vi "GFITS_getKeyvalueFromDBSHandler2.vi"(0 "key name in header":string, 1 "Database RefNum in":T3, 2 "action":enum16{"get", "clear"}(ring), 3 "extension":i32, 5 "varname":string, 7 "comment":string, 11 "error in (no error)":errorcluster, 12 "nd queue":bool, 13 "expID in":string) -> (6 "table out":string[][](table), 8 "expID":string, 10 "datatype":u16[](array[numeric]), 14 "function to use":string, 15 "error out":errorcluster)   [LabVIEW 2016]
uses:
  GFITS_datatypesctl.ctl
  DBSHAND/private/vis/DatabaseHand_RefNum.ctl
  DBSHAND/private/vis/DatabaseHand_Element_Get(3DArr).vi
  DBSHAND/private/vis/DatabaseHand_Element_Get(1DArr).vi
  DBSHAND/private/vis/DatabaseHand_Element_Get(string).vi
panel:
  out "Array":T1(array[cluster])
  in  "key":T2
  in  "Types":T4={"TBIT"=1, "TBYTE"=11, "TSTRING"=16, "TSHORT"=21, "TLONG"=41, "TFLOAT"=42, "TDOUBLE"=82, "TCOMPLEX"=83, "TDBLCOMPLEX"=163, "TUINT"=30, "TUSHORT"=20, "TULONG"=40, "TINT"=31, "TSBYTE"=12, "TLONGLONG"=81, "TLOGICAL"=14}
  in  "Supported DataTypes":i32(listbox)
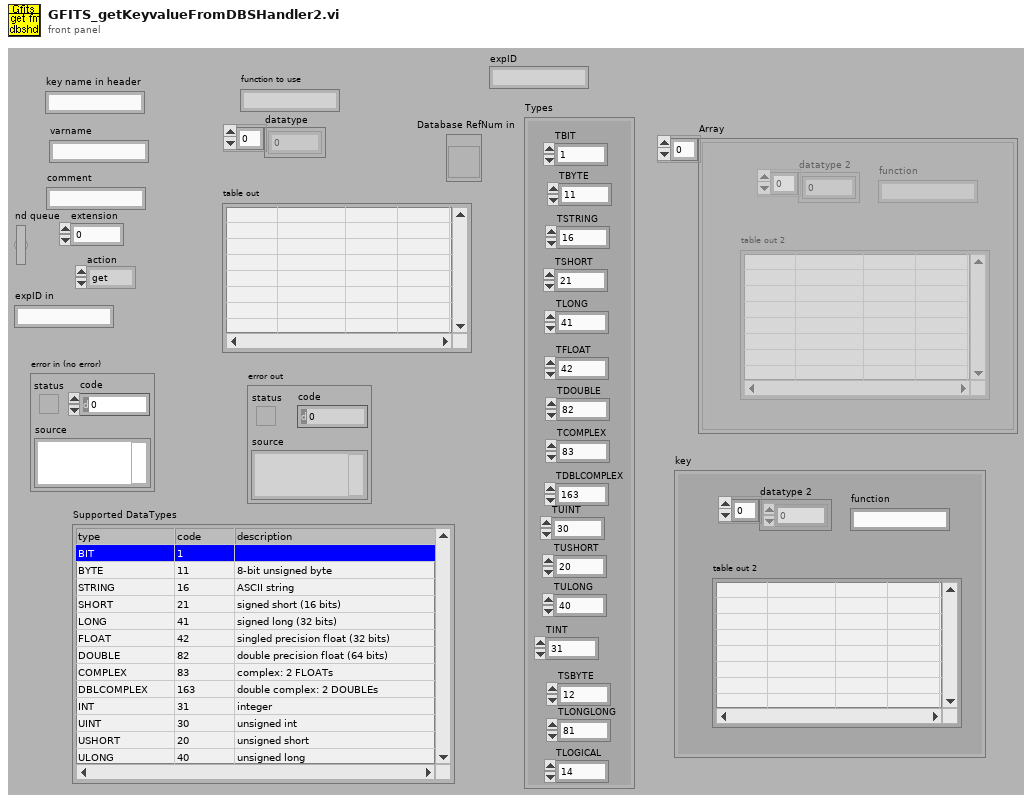
[diagram p1: front panel]
types:
  T1 = cluster{"table out 2":string[][], "datatype 2":u16[], "function":string}[]
  T2 = cluster{"table out 2":string[][], "datatype 2":u16[], "function":string}
  T3 = typedef "DatabaseHand_RefNum.ctl" = refnum<vi>
  T4 = typedef "GFITS_datatypesctl.ctl" = cluster{"TBIT":i32, "TBYTE":i32, "TSTRING":i32, "TSHORT":i32, "TLONG":i32, "TFLOAT":i32, "TDOUBLE":i32, "TCOMPLEX":i32, "TDBLCOMPLEX":i32, "TUINT":i32, "TUSHORT":i32, "TULONG":i32, "TINT":i32, "TSBYTE":i32, "TLONGLONG":i32, "TLOGICAL":i32}
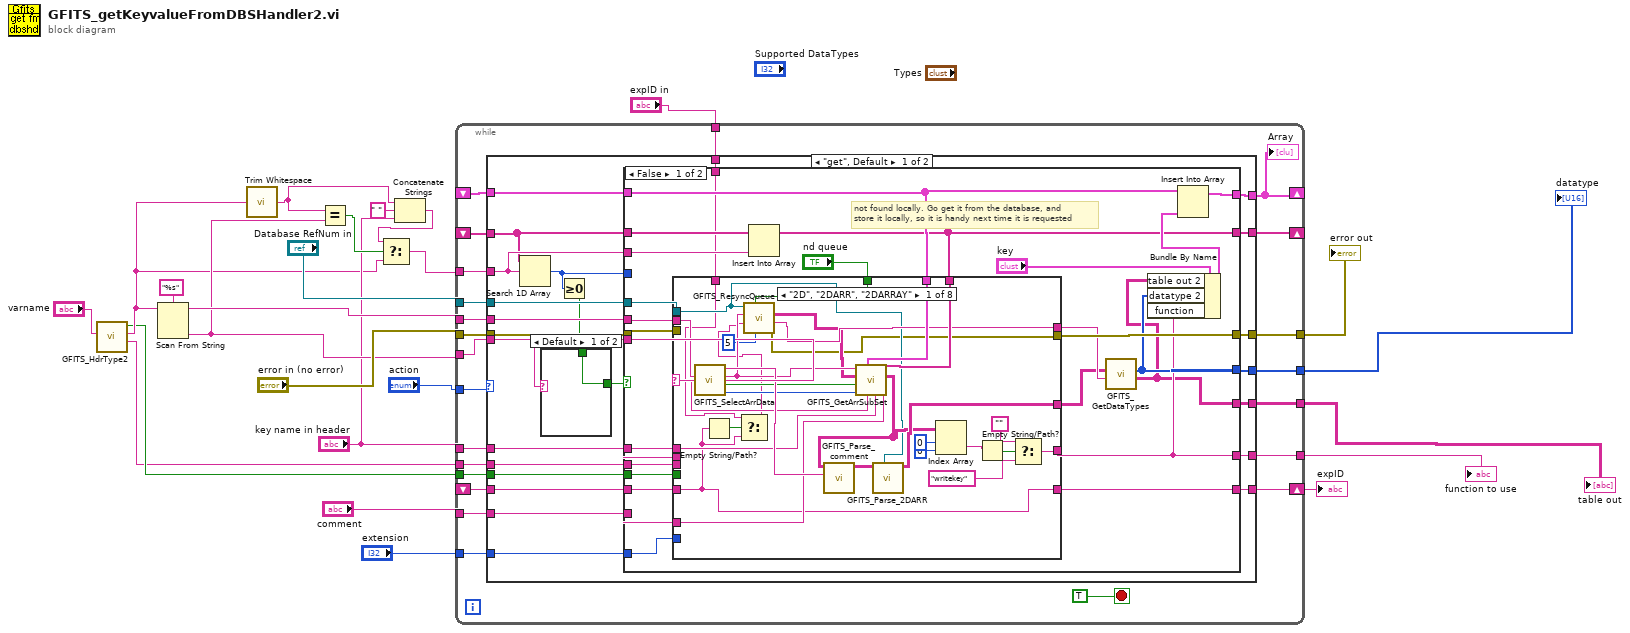
[diagram p0: block diagram]
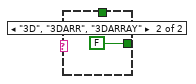
[diagram p2: hidden frame]
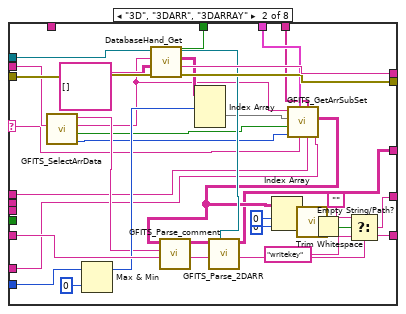
[diagram p3: hidden frame]
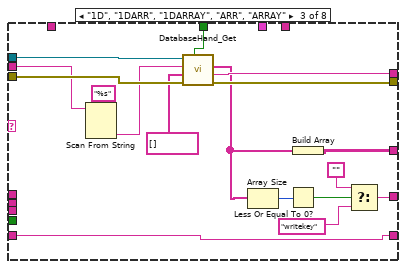
[diagram p4: hidden frame]
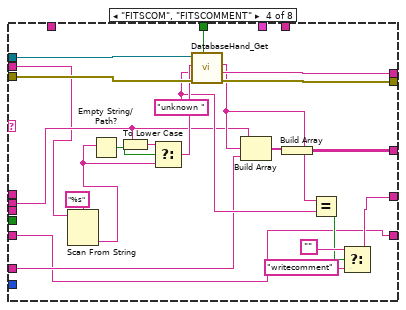
[diagram p5: hidden frame]
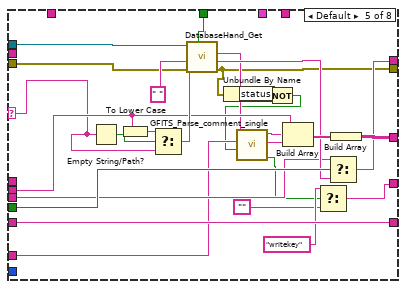
[diagram p6: hidden frame]
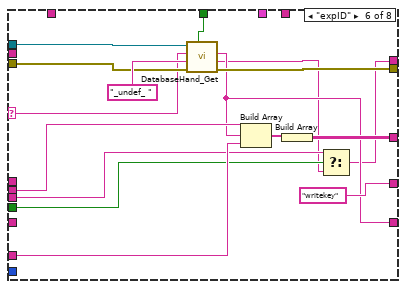
[diagram p7: hidden frame]
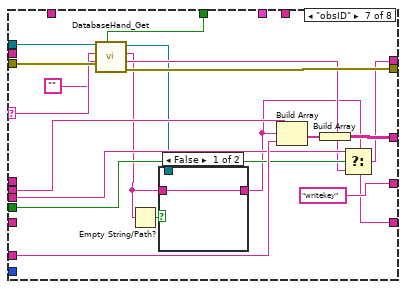
[diagram p8: hidden frame]
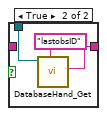
[diagram p9: hidden frame]
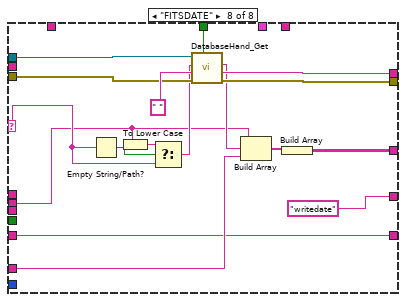
[diagram p10: hidden frame]
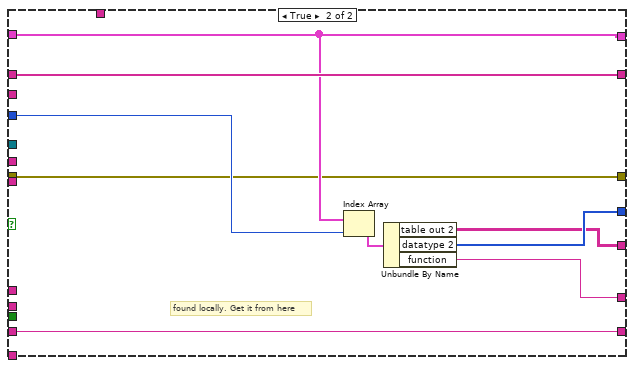
[diagram p11: hidden frame]
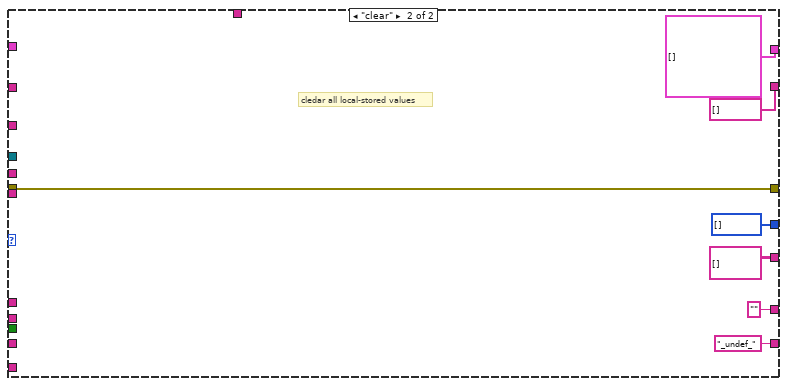
[diagram p12: hidden frame]
diagram:
  n1 = call "GFITS_HdrType2.vi"("keyval"="varname") -> ("type"=w2:string, "keyval out"=w4:string, "specified"=w3:bool)  [unwired: 8 out]
  n2 = Scan From String(format string="%s", input string=w4) -> (remaining string=w21:string, output 1=w14:string)  [unwired: 2 in, 3 out]
  n3 = call <vilib>:"Trim Whitespace.vi"("string"=w4) -> ("trimmed string"=w12:string)  [unwired: 1 in]
  n4 = Equal?(x=w12, y=w14) -> (x = y?=w13:bool)
  n5 = Concatenate Strings(w12, " " ("string"), "key name in header") -> (w9:string)
  n6 = Select(t=w9, s=w13, f=w4) -> (s? t:f=w8:string)
  n7 = while {
    tunnel: "Database RefNum in" -> [w47]
    tunnel: "error in (no error)" -> [w46]
    tunnel: w14 -> [w45]
    tunnel: w21 -> [w44]
    tunnel: [w43] -> w20
    tunnel: "key name in header" -> [w42]
    tunnel: "comment" -> [w41]
    tunnel: [w40] -> w19
    tunnel: [w39] -> w15
    shift-right: [w34] -> _
    shift-left: _ -> [w33]
    tunnel: "action" -> [w37]
    shift-right: [w31] -> _
    shift-left: _ -> [w32]
    tunnel: [w36] -> w17
    tunnel: w8 -> [w35]
    shift-right: [w30] -> w7
    shift-left: _ -> [w29]
    tunnel: "extension" -> [w28]
    tunnel: w3 -> [w27]
    tunnel: w2 -> [w26]
    tunnel: "expID in" -> [w25]
    stop <- TRUE stop-if-true
    n8 = case shown="\"get\", Default" w37 {
      tunnel: w47 -> [w71 _]
      tunnel: w46 -> [w70 w299]
      tunnel: w45 -> [w53 _]
      tunnel: w44 -> [w69 _]
      tunnel: [w68 "" ("function")] -> w43
      tunnel: w42 -> [w67 _]
      tunnel: w41 -> [w66 _]
      tunnel: [w65 w299] -> w40
      tunnel: [w64 string[][] []] -> w39
      tunnel: [w63 i32[] []] -> w36
      tunnel: w35 -> [w62 _]
      tunnel: [w61 string[] []] -> w34
      tunnel: [w60 T1 []] -> w31
      tunnel: w33 -> [w59 _]
      tunnel: w32 -> [w58 _]
      tunnel: [w56 "_undef_" ("value")] -> w30
      tunnel: w29 -> [w55 _]
      tunnel: w28 -> [w54 _]
      tunnel: w27 -> [w50 _]
      tunnel: w26 -> [w49 _]
      tunnel: w25 -> [w48 _]
      frame "get", Default {
        n9 = Search 1D Array(1D array=w59, element=w62) -> (index of element=w57:i32)  [unwired: 1 out]
        n10 = Greater Or Equal To 0?(x=w57) -> (x >= 0?=w52:bool)
        n11 = case shown="Default" w53 {
          tunnel: w52 -> [w72 _]
          tunnel: [w72 FALSE] -> w51
          frame Default {
          }
          frame "3D", "3DARR", "3DARRAY" {
          }
        }
        n12 = case shown="False" w51 {
          tunnel: w71 -> [w99 _]
          tunnel: w70 -> [w98 w288]
          tunnel: w69 -> [w97 _]
          tunnel: [w89 w289] -> w68
          tunnel: w67 -> [w75 _]
          tunnel: w66 -> [w96 _]
          tunnel: [w95 w288] -> w65
          tunnel: [w83 w287] -> w64
          tunnel: [w90 w290] -> w63
          tunnel: w53 -> [w93 _]
          tunnel: w62 -> [w80 _]
          tunnel: [w76 w294] -> w61
          tunnel: [w86 w293] -> w60
          tunnel: w59 -> [w88 w294]
          tunnel: w58 -> [w77 w293]
          tunnel: w57 -> [_ w292]
          tunnel: [w85 w286] -> w56
          tunnel: w55 -> [w84 w286]
          tunnel: w54 -> [w81 _]
          tunnel: w50 -> [w79 _]
          tunnel: w49 -> [w78 _]
          tunnel: w48 -> [w74 _]
          frame False {
            # "not found locally. Go get it from the database, and\nstore it locally, so it is handy next time it is requested"
            n13 = Insert Into Array(array=w88, new element=w80) -> (w76:string[])  [unwired: 1 in]
            n14 = case shown="\"2D\", \"2DARR\", \"2DARRAY\"" w93 {
              selector: w93 -> [w113 w135 _ _ w218 w236 w256 w277]
              tunnel: w99 -> [w105 w163 w180 w202 w228 w244 w264 w284]
              tunnel: w98 -> [_ w162 w179 w201 w227 w243 w263 w283]
              tunnel: [w107 w161 w178 w200 w215 w230 w251 w282] -> w94
              tunnel: w97 -> [w120 w141 w177 w186 _ _ _ _]
              tunnel: [w121 w139 w170 w198 w225 w241 w261 w280] -> w91
              tunnel: [w104 w153 w171 w197 w209 w240 w260 w279] -> w95
              tunnel: [w124 w154 w172 w193 w205 "writekey" "writekey" "writedate"] -> w89
              tunnel: w75 -> [_ _ _ w187 w221 w238 w258 w272]
              tunnel: w96 -> [w111 w132 _ w183 w212 w237 w257 w271]
              tunnel: [w102 w149 w165 w182 w220 w235 w247 w270] -> w85
              tunnel: w84 -> [w102 w149 w165 w182 w220 _ _ w270]
              tunnel: "nd queue" -> [w108 w148 w164 w181 w219 w234 w255 w269]
              tunnel: w81 -> [_ w147 _ _ _ _ _ _]
              tunnel: w79 -> [_ _ _ _ w217 w233 w254 _]
              tunnel: w78 -> [_ _ _ _ w214 w232 w253 _]
              tunnel: w77 -> [w115 w137 _ _ _ _ _ _]
              tunnel: w76 -> [w114 w136 _ _ _ _ _ _]
              tunnel: w75 -> [w112 w133 _ _ _ _ _ _]
              tunnel: w74 -> [w100 _ _ _ _ _ _ _]
              frame "2D", "2DARR", "2DARRAY" {
                n15 = call "GFITS_SelectArrData.vi"("arr name"=w120) -> ("index"=w116:i32, "subset?"=w117:bool, "name out"=w110:string, "comment"=w119:string)  [unwired: 7 out]
                n16 = Empty String/Path?(string/path=w102) -> (empty?=w103:bool)
                n17 = Select(t=w100, s=w103, f=w102) -> (s? t:f=w101:string)
                n18 = call "GFITS_ResyncQueue.vi"("maxtries"=5, "nd queue"=w108, "ID in"=w101, "var name"=w110, "RefNum in"=w105) -> ("error out"=w104:errorcluster, "str datatype"=w107:string, "value out"=w106:string[][])  [unwired: 4 out]
                n19 = call "GFITS_GetArrSubSet.vi"("newcom"=w111, "newkey"=w112, "stored names"=w114, "array type"=w113, "stored vals"=w115, "index"=w116, "subset?"=w117, "dbs table"=w106, "array name"=w110) -> ("arr subset"=w118:string[][])  [unwired: 2 out]
                n20 = call "GFITS_Parse_comment.vi"("comment in"=w119, "array in"=w118) -> ("array out"=w122:string[][])  [unwired: 9 out]
                n21 = call "GFITS_Parse_2DARR.vi"("Database RefNum in"=w105, "array in"=w122) -> ("array out"=w121:string[][])  [unwired: 9 out]
                n22 = Index Array(array=w118, index (row)=0, index (col)=0 ("disabled index (col)")) -> (element=w127:string)
                n23 = Empty String/Path?(string/path=w127) -> (empty?=w126:bool)
                n24 = Select(t="", s=w126, f="writekey") -> (s? t:f=w124:string)
              }
              frame "3D", "3DARR", "3DARRAY" {
                n25 = call "GFITS_SelectArrData.vi"("arr name"=w141) -> ("index"=w130:i32, "subset?"=w138:bool, "name out"=w134:string, "comment"=w140:string)  [unwired: 7 out]
                n26 = Max & Min(x=w147, y=0) -> (max(x,y)=w144:i32)  [unwired: 1 out]
                n27 = call-poly "DatabaseHand_Get.vi"("nd queue"=w148, "error in (no error)"=w162, "default value"=string[][][] [], "name"=w134, "Database RefNum in"=w163) -> ("error out"=w153:errorcluster, "type"=w161:string, "value"=w145:string[][][], "Database RefNum out"=w150:T3)  [unwired: 3 out]
                n28 = Index Array(array=w145, index (dim 0)=w144) -> (element=w131:string[][])  [unwired: 2 in]
                n29 = call "GFITS_GetArrSubSet.vi"("newcom"=w132, "newkey"=w133, "stored names"=w136, "array type"=w135, "stored vals"=w137, "index"=w130, "subset?"=w138, "dbs table"=w131, "array name"=w134) -> ("arr subset"=w143:string[][])  [unwired: 2 out]
                n30 = call "GFITS_Parse_comment.vi"("comment in"=w140, "array in"=w143) -> ("array out"=w151:string[][])  [unwired: 9 out]
                n31 = call "GFITS_Parse_2DARR.vi"("Database RefNum in"=w150, "array in"=w151) -> ("array out"=w139:string[][])  [unwired: 9 out]
                n32 = Index Array(array=w143, index (row)=0, index (col)=0 ("disabled index (col)")) -> (element=w157:string)
                n33 = call <vilib>:"Trim Whitespace.vi"("string"=w157) -> ("trimmed string"=w142:string)  [unwired: 1 in]
                n34 = Empty String/Path?(string/path=w142) -> (empty?=w156:bool)
                n35 = Select(t="", s=w156, f="writekey") -> (s? t:f=w154:string)
              }
              frame "1D", "1DARR", "1DARRAY", "ARR", "ARRAY" {
                n36 = Scan From String(format string="%s", input string=w177) -> (output 1=w175:string)  [unwired: 2 in, 4 out]
                n37 = call-poly "DatabaseHand_Get.vi"("nd queue"=w164, "error in (no error)"=w179, "default value"=string[] [], "name"=w175, "Database RefNum in"=w180) -> ("error out"=w171:errorcluster, "type"=w178:string, "value"=w169:string[])  [unwired: 4 out]
                n38 = Array Size(array=w169) -> (size(s)=w168:i32)
                n39 = Less Or Equal To 0?(x=w168) -> (x <= 0?=w167:bool)
                n40 = Build Array(w169) -> (w170:string[][])
                n41 = Select(t="", s=w167, f="writekey") -> (s? t:f=w172:string)
              }
              frame "FITSCOM", "FITSCOMMENT" {
                w188 = "unknown "
                n42 = Scan From String(format string="%s", input string=w186) -> (output 1=w184:string)  [unwired: 2 in, 4 out]
                n43 = Empty String/Path?(string/path=w184) -> (empty?=w196:bool)
                n44 = To Lower Case(string=w187) -> (all lower case string=w195:string)
                n45 = Select(t=w195, s=w196, f=w184) -> (s? t:f=w194:string)
                n46 = call-poly "DatabaseHand_Get.vi"("nd queue"=w181, "error in (no error)"=w201, "default value"=w188, "name"=w194, "Database RefNum in"=w202) -> ("error out"=w197:errorcluster, "type"=w200:string, "value"=w192:string)  [unwired: 4 out]
                n47 = Build Array(w187, w192, w183) -> (w199:string[])
                n48 = Build Array(w199) -> (w198:string[][])
                n49 = Equal?(x=w192, y=w188) -> (x = y?=w189:bool)
                n50 = Select(t="", s=w189, f="writecomment") -> (s? t:f=w193:string)
              }
              frame Default {
                n51 = Empty String/Path?(string/path=w218) -> (empty?=w224:bool)
                n52 = To Lower Case(string=w221) -> (all lower case string=w223:string)
                n53 = Select(t=w223, s=w224, f=w218) -> (s? t:f=w222:string)
                n54 = call-poly "DatabaseHand_Get.vi"("nd queue"=w219, "error in (no error)"=w227, "default value"=" ", "name"=w222, "Database RefNum in"=w228) -> ("error out"=w209:errorcluster, "type"=w216:string, "value"=w213:string)  [unwired: 4 out]
                n55 = Unbundle By Name(w209) -> ("status"=w208:bool)
                n56 = Not(x=w208) -> (.not. x?=w204:bool)
                n57 = call "GFITS_Parse_comment_single.vi"("found"=w204, "comment in"=w212, "value in"=w213) -> ("write?"=w206:bool, "comment out"=w210:string, "value out"=w211:string)  [unwired: 6 out]
                n58 = Build Array(w221, w211, w210) -> (w226:string[])
                n59 = Select(t="writekey", s=w206, f="") -> (s? t:f=w205:string)
                n60 = Select(t=w214, s=w217, f=w216) -> (s? t:f=w215:string)
                n61 = Build Array(w226) -> (w225:string[][])
              }
              frame "expID" {
                n62 = call-poly "DatabaseHand_Get.vi"("nd queue"=w234, "error in (no error)"=w243, "default value"="_undef_ ", "name"=w236, "Database RefNum in"=w244) -> ("error out"=w240:errorcluster, "type"=w231:string, "value"=w235:string)  [unwired: 4 out]
                n63 = Build Array(w238, w235, w237) -> (w242:string[])
                n64 = Build Array(w242) -> (w241:string[][])
                n65 = Select(t=w232, s=w233, f=w231) -> (s? t:f=w230:string)
              }
              frame "obsID" {
                n66 = call-poly "DatabaseHand_Get.vi"("nd queue"=w255, "error in (no error)"=w263, "default value"="", "name"=w256, "Database RefNum in"=w264) -> ("error out"=w260:errorcluster, "type"=w252:string, "value"=w248:string, "Database RefNum out"=w250:T3)  [unwired: 3 out]
                n67 = Empty String/Path?(string/path=w248) -> (empty?=w249:bool)
                n68 = case shown="False" w249 {
                  tunnel: w250 -> [_ w267]
                  tunnel: w248 -> [w265 _]
                  tunnel: [w265 w266] -> w247
                  frame False {
                  }
                  frame True {
                    n69 = call-poly "DatabaseHand_Get.vi"("name"="lastobsID", "Database RefNum in"=w267) -> ("value"=w266:string)  [unwired: 3 in, 6 out]
                  }
                }
                n70 = Build Array(w258, w247, w257) -> (w262:string[])
                n71 = Build Array(w262) -> (w261:string[][])
                n72 = Select(t=w253, s=w254, f=w252) -> (s? t:f=w251:string)
              }
              frame "FITSDATE" {
                n73 = Empty String/Path?(string/path=w277) -> (empty?=w278:bool)
                n74 = To Lower Case(string=w272) -> (all lower case string=w276:string)
                n75 = Select(t=w276, s=w278, f=w277) -> (s? t:f=w275:string)
                n76 = call-poly "DatabaseHand_Get.vi"("nd queue"=w269, "error in (no error)"=w283, "default value"=" ", "name"=w275, "Database RefNum in"=w284) -> ("error out"=w279:errorcluster, "type"=w282:string, "value"=w273:string)  [unwired: 4 out]
                n77 = Build Array(w272, w273, w271) -> (w281:string[])
                n78 = Build Array(w281) -> (w280:string[][])
              }
            }
            n79 = call "GFITS_GetDataTypes.vi"("type"=w94, "keys"=w91) -> ("keys out"=w83:string[][], "datatypes"=w90:i32[])  [unwired: 8 out]
            n80 = Bundle By Name(cluster="key", "table out 2"=w83, "datatype 2"=w90, "function"=w89) -> (w87:T2)
            n81 = Insert Into Array(array=w77, new element=w87) -> (w86:T1)  [unwired: 1 in]
          }
          frame True {
            # "found locally. Get it from here"
            n82 = Index Array(array=w293, index=w292) -> (element=w291:T2)
            n83 = Unbundle By Name(w291) -> ("table out 2"=w287:string[][], "datatype 2"=w290:u16[], "function"=w289:string)
          }
        }
      }
      frame "clear" {
        # "cledar all local-stored values"
      }
    }
    "Array" <- w31
  }
  "datatype" <- w17
  "function to use" <- w20
  "table out" <- w15
  "error out" <- w19
  "expID" <- w7
